vi "Pre Launch Init.vi"(11 "Camera_Prime95B in":refnum<class "Camera_Prime95B.lvclass">) -> (0 "error out":errorcluster, 3 "Camera_Prime95B out":refnum<class "Camera_Prime95B.lvclass">)   [LabVIEW 2020, in "Camera_Prime95B.lvlib" / "Camera_Prime95B.lvclass"]
doc: "(<B>Filename</B>: Actor Framework.lvlib:Actor.lvclass:Pre Launch Init.vi)\n\nDefines behavior that occurs after the Launch Nested Actor method is invoked but before the actor's Actor Core method begins running.\n\nBy default, this method does nothing. A descendant class may override it to define behavior."
uses:
  Camera_Prime95B.lvclass
  HAL Layer/Camera/Camera/Camera.lvclass
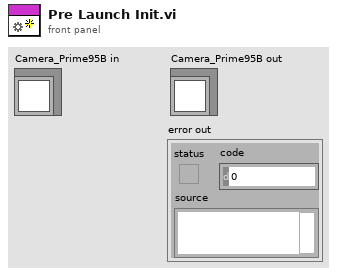
[diagram p1: front panel]
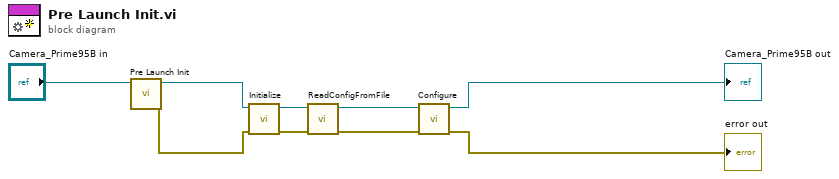
[diagram p0: block diagram]
diagram:
  n1 = call-parent "Pre Launch Init.vi"("Device in"="Camera_Prime95B in") -> ("error out"=w6:errorcluster, "Device out"=w2:refnum<class "Camera_Prime95B.lvclass">)  [unwired: 9 in]
  n2 = call-dynamic "Initialize.vi"("error in (no error)"=w6, "Camera_Prime95B in"=w2) -> ("error out"=w7:errorcluster, "Camera_Prime95B out"=w4:refnum<class "Camera_Prime95B.lvclass">)  [unwired: 8 in]
  n3 = call-dynamic "ReadConfigFromFile.vi"("error in (no error)"=w7, "Camera_Prime95B in"=w4) -> ("error out"=w8:errorcluster, "Camera_Prime95B out"=w3:refnum<class "Camera_Prime95B.lvclass">)  [unwired: 8 in]
  n4 = call-dynamic "Configure.vi"("error in (no error)"=w8, "Camera_Prime95B in"=w3) -> ("error out"=→"error out":errorcluster, "Camera_Prime95B out"=→"Camera_Prime95B out":refnum<class "Camera_Prime95B.lvclass">)  [unwired: 8 in]
